vi "Begin.vi"(8 "error in":errorcluster) -> (0 "error out":errorcluster)   [LabVIEW 2023]
doc: "Called before other user functions, this VI is expected to open initial I/O refnums, load in file data, and do all program initialization. Notice that the <B>error out</B> terminal is simply used for data flow. Wiring it to other structures or subVIs ensures that this VI runs first."
uses:
  <vilib>/Rock Robotics/WPI/DriverStation/WPI_DriverStationRobotMode2.ctl
  <vilib>/Rock Robotics/WPI/Joystick/WPI_JoystickDeviceEnum.ctl
  <vilib>/Rock Robotics/WPI/ThirdParty/REV Robotics/REVLib/Typedef/Spark MAX Control Type.ctl
  <vilib>/Rock Robotics/WPI/ThirdParty/REV Robotics/REVLib/Typedef/Spark MAX Limit Direction.ctl
  <vilib>/Rock Robotics/WPI/ThirdParty/REV Robotics/REVLib/Typedef/Spark MAX Limit Switch Polarity.ctl
  <vilib>/Rock Robotics/WPI/Solenoid/WPI_SolenoidChannel.ctl
  <vilib>/Rock Robotics/WPI/Solenoid/WPI_SolenoidValue.ctl
  <vilib>/Rock Robotics/SystemInterfaces/DIO/FPGA_DIOChannel.ctl
  Robot Global Data.vi
  <vilib>/Rock Robotics/Network Tables/NT Write String Array.vi
  <vilib>/Rock Robotics/WPI/Utilities/WPI_GetSetVariantRefNum.vi
  <vilib>/Rock Robotics/WPI/Solenoid/WPI_SolenoidOpenDouble.vi
  <vilib>/Rock Robotics/WPI/Solenoid/WPI_SolenoidSetEnum.vi
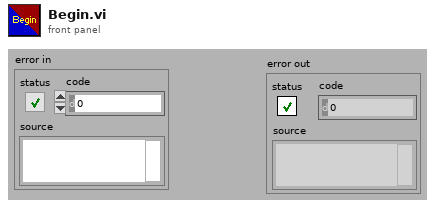
[diagram p1: front panel]
types:
  T1 = typedef "FPGA_DIOChannel.ctl" = enum8{"DIO 0", "DIO 1", "DIO 2", "DIO 3", "DIO 4", "DIO 5", "DIO 6", "DIO 7", "DIO 8", "DIO 9", "DIO MXP 0", "DIO MXP 1", "DIO MXP 2", "DIO MXP 3", "DIO MXP 4", "DIO MXP 5", "DIO MXP 6", "DIO MXP 7", "DIO MXP 8", "DIO MXP 9", "DIO MXP 10", "DIO MXP 11", "DIO MXP 12", "DIO MXP 13", "DIO MXP 14", "DIO MXP 15", "SPI Port CS1", "SPI Port CS2", "SPI Port CS3", "SPI Port MISO", "SPI Port MOSI", "Invalid"}
  T2 = typedef "WPI_SolenoidValue.ctl" = enum16{"Off", "On", "Forward", "Reverse"}
  T3 = typedef "WPI_SolenoidChannel.ctl" = enum8{"Solenoid 0", "Solenoid 1", "Solenoid 2", "Solenoid 3", "Solenoid 4", "Solenoid 5", "Solenoid 6", "Solenoid 7", "Solenoid 8", "Solenoid 9", "Solenoid 10", "Solenoid 11", "Solenoid 12", "Solenoid 13", "Solenoid 14", "Solenoid 15", "Invalid"}
  T4 = typedef "Spark MAX Limit Direction.ctl" = enum16{"Forward Limit", "Reverse Limit"}
  T5 = typedef "Spark MAX Limit Switch Polarity.ctl" = enum16{"Normally Open", "Normally Closed"}
  T6 = typedef "Spark MAX Control Type.ctl" = enum16{"Percent VBus", "Voltage", "Velocity", "Position", "Smart Motion", "Current", "Smart Velocity"}
  T7 = typedef "WPI_JoystickDeviceEnum.ctl" = enum16{"USB 0", "USB 1", "USB 2", "USB 3", "USB 4", "USB 5"}
  T8 = typedef "WPI_DriverStationRobotMode2.ctl" = enum16{"Autonomous Disabled", "Autonomous Enabled", "Teleop Disabled", "Teleop Enabled", "Disconnected", "Finish", "Test Disabled", "Test Enabled", "Emergency Stopped"}
  T9 = typedef "WPI_MotorControlDeviceRef.ctl" = cluster{"DeviceStatus":errorcluster, "Type":T10, "PWM":cluster{"PWM Channel":T11, "DeadBand":T12}, "CAN":cluster{"Device Number":u8, "SetOutput VI Ref":variant, "GetOutput VI Ref":variant, "Enable VI Ref":variant, "Disable VI Ref":variant, "Data":variant}, "Invert":bool, "DIO PWM":cluster{"PWM \"Enable\" Channel":T11, "DIOChannel":T1, "PWM Rate":dbl}}
  T10 = typedef "WPI_MotorControlType.ctl" = enum16{"PWM", "CAN", "DIO PWM"}
  T11 = typedef "FPGA_DIOPWMChannel.ctl" = enum8{"PWM 0", "PWM 1", "PWM 2", "PWM 3", "PWM 4", "PWM 5", "PWM 6", "PWM 7", "PWM 8", "PWM 9", "PWM MXP 0", "PWM MXP 1", "PWM MXP 2", "PWM MXP 3", "PWM MXP 4", "PWM MXP 5", "PWM MXP 6", "PWM MXP 7", "PWM MXP 8", "PWM MXP 9", "Invalid"}
  T12 = typedef "WPI_PWMDeadband.ctl" = cluster{"Name":string, "maxPositivePwm":i32, "minPositivePwm":i32, "centerPwm":i32, "maxNegativePwm":i32, "minNegativePwm":i32, "angularRange":u16}
  T13 = typedef "WPI_DigitalInputDevRef.ctl" = cluster{"DevStatus":errorcluster, "DIO Channel":T1}
  T14 = typedef "WPI_JoystickDevRef.ctl" = cluster{"Device":T7}
  T15 = typedef "WPI_SolenoidDevRef.ctl" = cluster{"DevStatus":errorcluster, "Pneumatics Control Module":u8, "Forward Solenoid Channel":T3, "Reverse Solenoid Channel":T3}
  T16 = typedef "WPI_CompressorDevRef.ctl" = cluster{"DevStatus":errorcluster, "Pneumatics Control Module":u8}
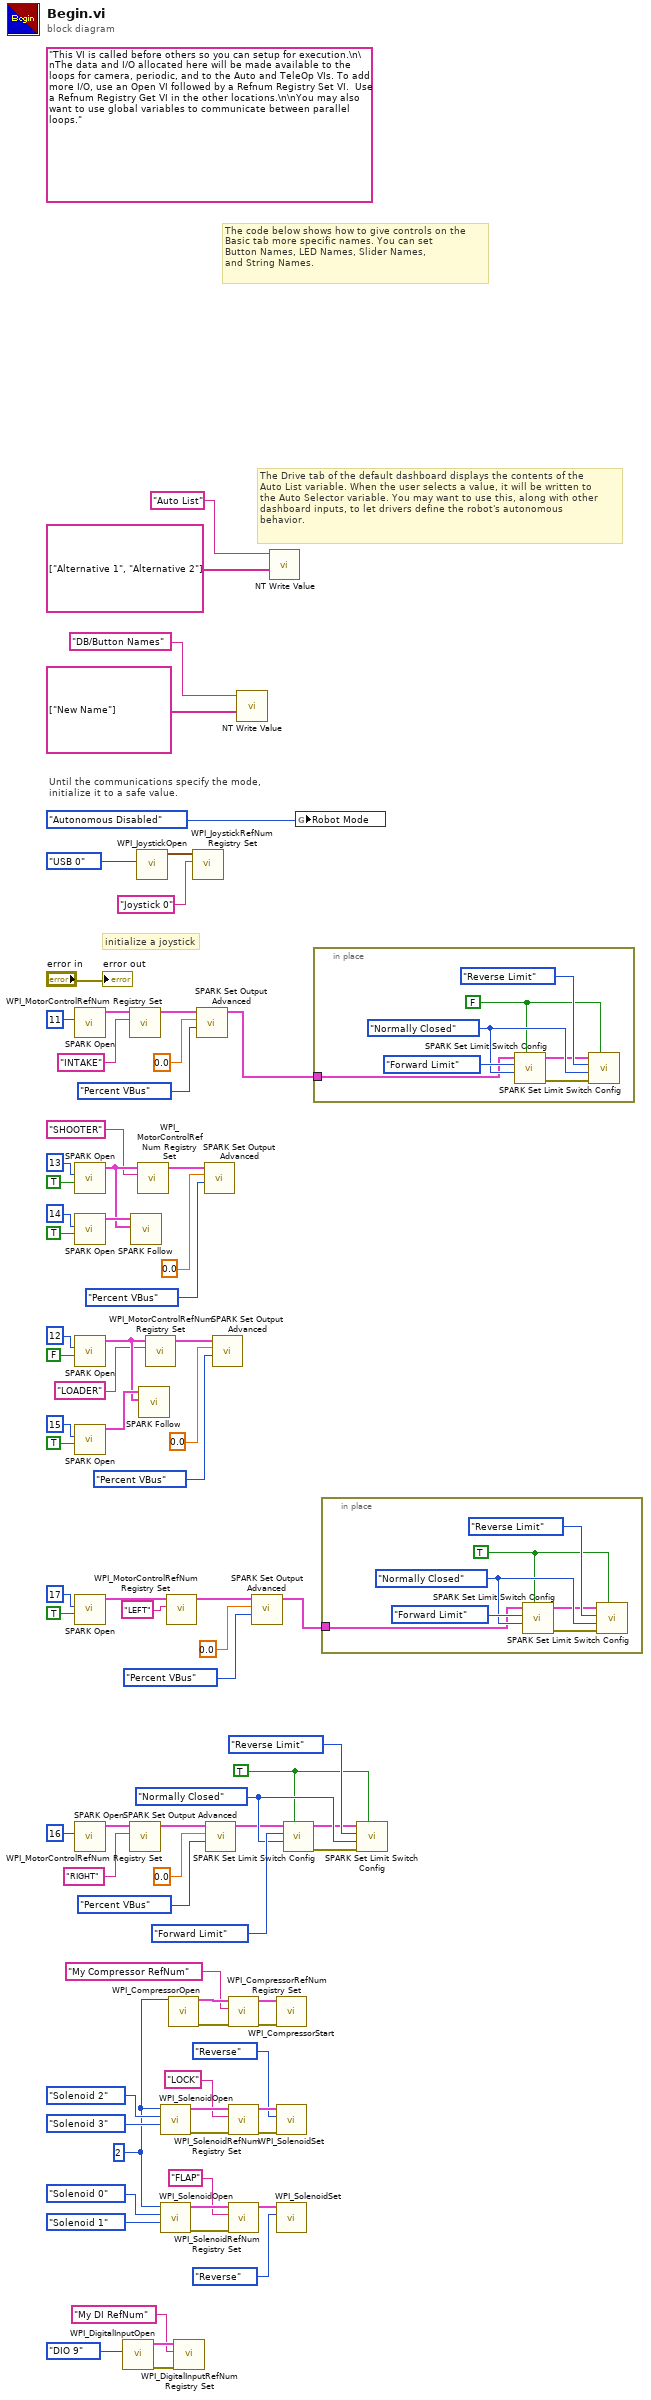
[diagram p0: block diagram]
diagram:
  w12 = u8 2 ("Pneumatics device (def)")
  w30 = TRUE ("Enabled? (T)")
  w34 = Spark_MAX_Limit_Switch_Polarity."Normally Closed" ("Polarity (Normally Open)")
  (unwired) "This VI is called before others so you can setup for execution.\n\nThe data and I/O allocated here will be made available to the loops for camera, periodic, and to the Auto and TeleOp VIs. To add more I/O, use an Open VI followed by a Refnum Registry Set VI.  Use a Refnum Registry Get VI in the other locations.\n\nYou may also want to use global variables to communicate between parallel loops."
  # "The Drive tab of the default dashboard displays the contents of the\nAuto List variable. When the user selects a value, it will be written to\nthe Auto Selector variable. You may want to use this, along with other\ndashboard inputs, to let drivers define the robot's autonomous\nbehavior."
  # "The code below shows how to give controls on the\nBasic tab more specific names. You can set\nButton Names, LED Names, Slider Names,\nand String Names."
  # "initialize a joystick"
  # "Until the communications specify the mode,\ninitialize it to a safe value."
  n1 = call <vilib>:"SPARK Open.vi"("Device Number"=u8 11) -> ("MotorControlDeviceRef"=w61:T9)  [unwired: 9 in, 1 out]
  n2 = call <vilib>:"SPARK Open.vi"("Invert"=TRUE, "Device Number"=u8 13) -> ("MotorControlDeviceRef"=w56:T9)  [unwired: 8 in, 1 out]
  n3 = call <vilib>:"SPARK Open.vi"("Invert"=TRUE, "Device Number"=u8 14) -> ("MotorControlDeviceRef"=w57:T9)  [unwired: 8 in, 1 out]
  n4 = call <vilib>:"SPARK Open.vi"("Invert"=FALSE, "Device Number"=u8 12) -> ("MotorControlDeviceRef"=w69:T9)  [unwired: 8 in, 1 out]
  n5 = call <vilib>:"SPARK Open.vi"("Invert"=TRUE, "Device Number"=u8 15) -> ("MotorControlDeviceRef"=w70:T9)  [unwired: 8 in, 1 out]
  n6 = call <vilib>:"SPARK Open.vi"("Invert"=TRUE, "Device Number"=u8 17) -> ("MotorControlDeviceRef"=w45:T9)  [unwired: 8 in, 1 out]
  n7 = call <vilib>:"SPARK Open.vi"("Device Number"=u8 16) -> ("MotorControlDeviceRef"=w39:T9)  [unwired: 9 in, 1 out]
  n8 = call <vilib>:"WPI_DigitalInputOpen.vi"("DIO Channel"=FPGA_DIOChannel."DIO 9") -> ("error out"=w4:errorcluster, "DigitalInputDevRef"=w3:T13)  [unwired: 9 in]
  n9 = call <vilib>:"WPI_MotorControlRefNum Registry Set.vi"("refnum name"="INTAKE", "MotorControlDevRef"=w61) -> ("MotorControlDevRef"=w64:T9)  [unwired: 8 in, 1 out]
  n10 = call <vilib>:"WPI_MotorControlRefNum Registry Set.vi"("refnum name"="RIGHT", "MotorControlDevRef"=w39) -> ("MotorControlDevRef"=w42:T9)  [unwired: 8 in, 1 out]
  n11 = call <vilib>:"SPARK Follow.vi"("Master Controller"=w56, "MotorControlDeviceRef"=w57) -> ()  [unwired: 8 in, 2 out]
  n12 = call <vilib>:"WPI_JoystickOpen.vi"("JoystickDevice"=WPI_JoystickDeviceEnum."USB 0") -> ("JoystickDevRef"=w80:T14)  [unwired: 10 in]
  n13 = call <vilib>:"WPI_MotorControlRefNum Registry Set.vi"("refnum name"="SHOOTER", "MotorControlDevRef"=w56) -> ("MotorControlDevRef"=w54:T9)  [unwired: 8 in, 1 out]
  n14 = call <vilib>:"SPARK Follow.vi"("Master Controller"=w69, "MotorControlDeviceRef"=w70) -> ()  [unwired: 8 in, 2 out]
  n15 = call <vilib>:"WPI_MotorControlRefNum Registry Set.vi"("refnum name"="LOADER", "MotorControlDevRef"=w69) -> ("MotorControlDevRef"=w67:T9)  [unwired: 8 in, 1 out]
  n16 = call-poly <vilib>:"WPI_SolenoidOpen.vi"("Reverse Solenoid Channel"=WPI_SolenoidChannel."Solenoid 3", "Forward Solenoid Channel"=WPI_SolenoidChannel."Solenoid 2", "Pneumatics Device (def)"=w12) -> ("error out"=w15:errorcluster, "SolenoidDevRef"=w14:T15)  [unwired: 7 in]
  n17 = call-poly <vilib>:"WPI_SolenoidOpen.vi"("Reverse Solenoid Channel"=WPI_SolenoidChannel."Solenoid 1", "Forward Solenoid Channel"=WPI_SolenoidChannel."Solenoid 0", "Pneumatics Device (def)"=w12) -> ("error out"=w20:errorcluster, "SolenoidDevRef"=w19:T15)  [unwired: 7 in]
  n18 = call <vilib>:"WPI_MotorControlRefNum Registry Set.vi"("refnum name"="LEFT", "MotorControlDevRef"=w45) -> ("MotorControlDevRef"=w48:T9)  [unwired: 8 in, 1 out]
  n19 = call <vilib>:"WPI_CompressorOpen.vi"("Pneumatics device (def)"=w12) -> ("CompressorDevRef"=w26:T16, "error out"=w27:errorcluster)  [unwired: 13 in]
  n20 = call <vilib>:"WPI_DigitalInputRefNum Registry Set.vi"("error in (no error)"=w4, "refnum name"="My DI RefNum", "DigitalInputDevRef"=w3) -> ()  [unwired: 7 in, 2 out]
  n21 = call <vilib>:"WPI_JoystickRefNum Registry Set.vi"("refnum name"="Joystick 0", "JoystickDevRef"=w80) -> ()  [unwired: 8 in, 2 out]
  n22 = call <vilib>:"SPARK Set Output Advanced.vi"("Control Mode"=Spark_MAX_Control_Type."Percent VBus", "Setpoint"=0.0 ("Output"), "MotorControlDevRef"=w64) -> ("MotorControlDevRef"=w1:T9)  [unwired: 7 in, 1 out]
  n23 = call <vilib>:"SPARK Set Output Advanced.vi"("Control Mode"=Spark_MAX_Control_Type."Percent VBus", "Setpoint"=0.0 ("Output"), "MotorControlDevRef"=w54) -> ()  [unwired: 7 in, 2 out]
  n24 = call <vilib>:"SPARK Set Output Advanced.vi"("Control Mode"=Spark_MAX_Control_Type."Percent VBus", "Setpoint"=0.0 ("Output"), "MotorControlDevRef"=w42) -> ("MotorControlDevRef"=w29:T9)  [unwired: 7 in, 1 out]
  n25 = call <vilib>:"SPARK Set Output Advanced.vi"("Control Mode"=Spark_MAX_Control_Type."Percent VBus", "Setpoint"=0.0 ("Output"), "MotorControlDevRef"=w67) -> ()  [unwired: 7 in, 2 out]
  n26 = call <vilib>:"WPI_CompressorRefNum Registry Set.vi"("error in (no error)"=w27, "refnum name"="My Compressor RefNum", "CompressorDevRef"=w26) -> ("error out"=w24:errorcluster, "CompressorDevRef"=w23:T16)  [unwired: 7 in]
  n27 = call <vilib>:"WPI_SolenoidRefNum Registry Set.vi"("error in (no error)"=w15, "refnum name"="LOCK", "SolenoidDevRef"=w14) -> ("error out"=w11:errorcluster, "SolenoidDevRef"=w10:T15)  [unwired: 7 in]
  n28 = call <vilib>:"WPI_SolenoidRefNum Registry Set.vi"("error in (no error)"=w20, "refnum name"="FLAP", "SolenoidDevRef"=w19) -> ("SolenoidDevRef"=w8:T15)  [unwired: 7 in, 1 out]
  n29 = call-poly <vilib>:"NT Write Value.vi"("value"=string[] ["New Name"], "name"="DB/Button Names" ("Name")) -> ()  [unwired: 9 in, 1 out]
  n30 = call <vilib>:"SPARK Set Output Advanced.vi"("Control Mode"=Spark_MAX_Control_Type."Percent VBus", "Setpoint"=0.0 ("Output"), "MotorControlDevRef"=w48) -> ("MotorControlDevRef"=w28:T9)  [unwired: 7 in, 1 out]
  n31 = call-poly <vilib>:"NT Write Value.vi"("value"=string[] ["Alternative 1", "Alternative 2"] ("String Array"), "name"="Auto List" ("Name")) -> ()  [unwired: 9 in, 1 out]
  n32 = call <vilib>:"WPI_CompressorStart.vi"("error in (no error)"=w24, "CompressorDevRef"=w23) -> ()  [unwired: 8 in, 2 out]
  n33 = call-poly <vilib>:"WPI_SolenoidSet.vi"("error in (no error)"=w11, "Value"=WPI_SolenoidValue."Reverse", "SolenoidDevRef"=w10) -> ()  [unwired: 7 in, 2 out]
  n34 = call-poly <vilib>:"WPI_SolenoidSet.vi"("Value"=WPI_SolenoidValue."Reverse", "SolenoidDevRef"=w8) -> ()  [unwired: 8 in, 2 out]
  n35 = call <vilib>:"SPARK Set Limit Switch Config.vi"("Enabled? (T)"=w30, "Polarity (Normally Open)"=w34, "Limit Switch"=Spark_MAX_Limit_Direction."Forward Limit", "MotorControlDeviceRef in"=w29) -> ("error out"=w32:errorcluster, "MotorControlDeviceRef out"=w31:T9)  [unwired: 6 in]
  n36 = global write "Robot Global Data.vi" "Robot Mode"(WPI_DriverStationRobotMode2."Autonomous Disabled" ("Robot Mode")) -> ()
  n37 = in-place {
    in-place-border: w1 -> [w83]
    w84 = FALSE ("Enabled? (T)")
    w88 = Spark_MAX_Limit_Switch_Polarity."Normally Closed" ("Polarity (Normally Open)")
    n38 = call <vilib>:"SPARK Set Limit Switch Config.vi"("Enabled? (T)"=w84, "Polarity (Normally Open)"=w88, "Limit Switch"=Spark_MAX_Limit_Direction."Forward Limit", "MotorControlDeviceRef in"=w83) -> ("error out"=w86:errorcluster, "MotorControlDeviceRef out"=w85:T9)  [unwired: 6 in]
    n39 = call <vilib>:"SPARK Set Limit Switch Config.vi"("Enabled? (T)"=w84, "error in (no error)"=w86, "Polarity (Normally Open)"=w88, "Limit Switch"=Spark_MAX_Limit_Direction."Reverse Limit", "MotorControlDeviceRef in"=w85) -> ()  [unwired: 5 in, 2 out]
  }
  n40 = in-place {
    in-place-border: w28 -> [w90]
    w91 = TRUE ("Enabled? (T)")
    w95 = Spark_MAX_Limit_Switch_Polarity."Normally Closed" ("Polarity (Normally Open)")
    n41 = call <vilib>:"SPARK Set Limit Switch Config.vi"("Enabled? (T)"=w91, "Polarity (Normally Open)"=w95, "Limit Switch"=Spark_MAX_Limit_Direction."Forward Limit", "MotorControlDeviceRef in"=w90) -> ("error out"=w93:errorcluster, "MotorControlDeviceRef out"=w92:T9)  [unwired: 6 in]
    n42 = call <vilib>:"SPARK Set Limit Switch Config.vi"("Enabled? (T)"=w91, "error in (no error)"=w93, "Polarity (Normally Open)"=w95, "Limit Switch"=Spark_MAX_Limit_Direction."Reverse Limit", "MotorControlDeviceRef in"=w92) -> ()  [unwired: 5 in, 2 out]
  }
  n43 = call <vilib>:"SPARK Set Limit Switch Config.vi"("Enabled? (T)"=w30, "error in (no error)"=w32, "Polarity (Normally Open)"=w34, "Limit Switch"=Spark_MAX_Limit_Direction."Reverse Limit", "MotorControlDeviceRef in"=w31) -> ()  [unwired: 5 in, 2 out]
  "error out" <- "error in"
